vi "ParallelExecutionGlobal.vi"() -> ()   [LabVIEW 2020]
panel:
  out "DoMathsUsed":dbl
  out "loadRFPused":dbl
  in  "DoChannelMathsStrands":i32(slide) scale=-1.0..16.0
  in  "LoadRFPstrands":i32(slide) scale=-1.0..16.0
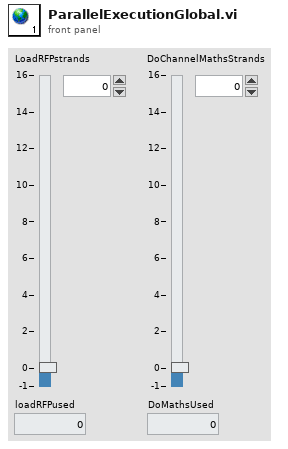
[diagram p1: front panel]
diagram:
